vi "BoxPath.vi"(10 "Path":path) -> (2 "Path out":refnum<class "Path.lvclass">)   [LabVIEW 2013, in "LapDog.Collections.v_.Common.lvlib" / "Path.lvclass"]
uses:
  Path.lvclass
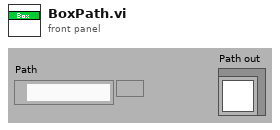
[diagram p1: front panel]
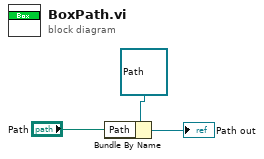
[diagram p0: block diagram]
diagram:
  n1 = Bundle By Name(cluster=refnum<class "Path.lvclass"> refnum ("LapDog.Collections.v0.Lists.Interfaces.lvlib:String.lvclass"), "Path"="Path") -> (→"Path out":refnum<class "Path.lvclass">)
